vi "SCMP - Populate preset cbk ring.vi"(8 "error in (no error)":errorcluster, 11 "preset cbk ring ref":refnum<vi>) -> (0 "error out":errorcluster)   [LabVIEW 2014]
doc: "Use this template to build a VI to use as a subVI."
panel:
  out "filenames":string[](array[string])
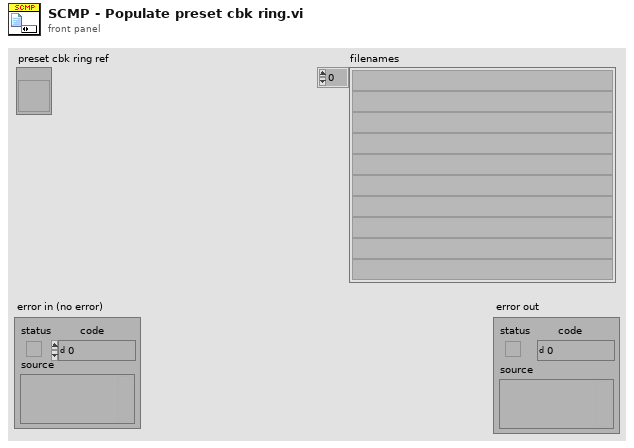
[diagram p1: front panel]
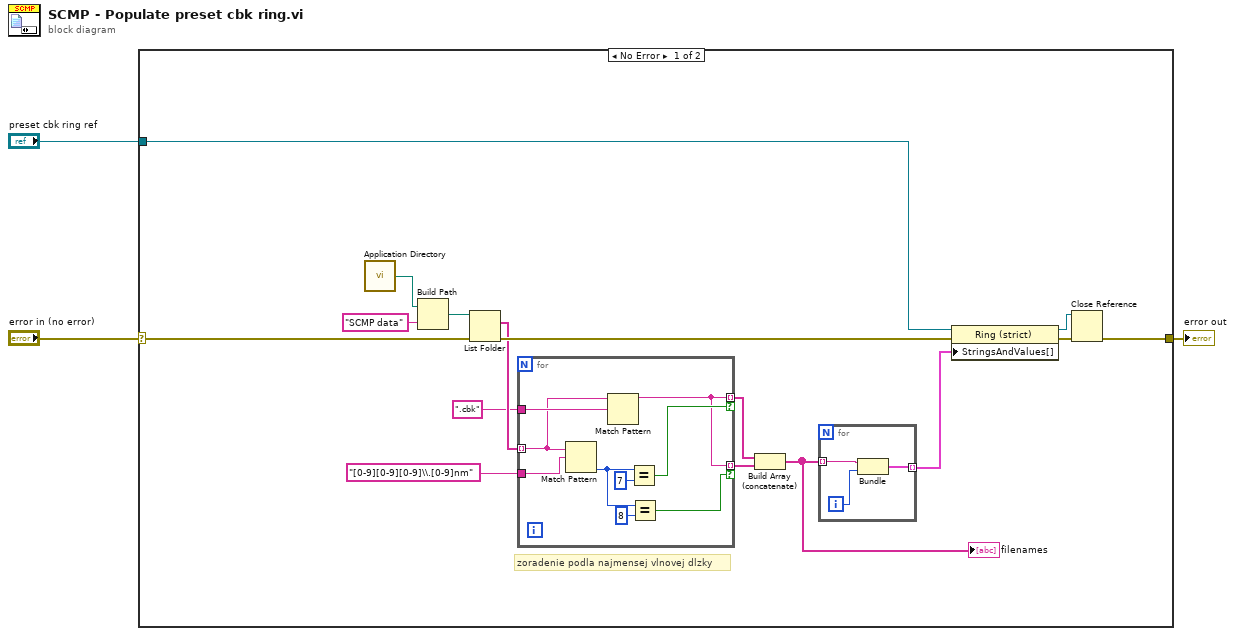
[diagram p0: block diagram]
diagram:
  n1 = case shown="No Error" "error in (no error)" {
    selector: "error in (no error)" -> [w18 w32]
    tunnel: [w15 w32] -> w2
    tunnel: "preset cbk ring ref" -> [w13 _]
    frame No Error {
      # "zoradenie podla najmensej vlnovej dlzky"
      n2 = call <vilib>:"Application Directory.vi"() -> ("Application Directory"=w12:path)
      n3 = Build Path(base path=w12, name or relative path="SCMP data") -> (appended path=w11:path)
      n4 = List Folder(path=w11, error in=w18) -> (filenames=w10:string[], error out=w17:errorcluster)  [unwired: 2 in, 2 out]
      n5 = for {
        tunnel: w10 -> [w24] mode=indexing
        tunnel: "[0-9][0-9][0-9]\\.[0-9]nm" ("pattern") -> [w30]
        tunnel: [w23] -> w8 mode=indexing if=w29
        tunnel: [w23] -> w7 mode=indexing if=w26
        tunnel: ".cbk" ("pattern") -> [w25]
        n6 = Match Pattern(string=w24, regular expression=w30) -> (offset past match=w27:i32)  [unwired: 1 in, 3 out]
        n7 = Match Pattern(string=w24, regular expression=w25) -> (before substring=w23:string)  [unwired: 1 in, 3 out]
        n8 = Equal?(x=w27, y=7) -> (x = y?=w29:bool)
        n9 = Equal?(x=w27, y=8) -> (x = y?=w26:bool)
      }
      n10 = Build Array (concatenate)(w8, w7) -> (w6:string[])
      "filenames" <- w6
      n11 = for {
        tunnel: w6 -> [w22] mode=indexing
        tunnel: [w20] -> w5 mode=indexing
        i -> [w21]
        n12 = Bundle(w22, w21) -> (w20:cluster{string, i32})  [unwired: 1 in]
      }
      n13 = property on="Property Node" class="Ring (strict)"(reference=w13, error in=w17, "StringsAndValues[]"=w5) -> (reference out=w14:refnum<vi>, error out=w16:errorcluster)
      n14 = Close Reference(reference=w14, error in (no error)=w16) -> (error out=w15:errorcluster)
    }
    frame Error {
    }
  }
  "error out" <- w2
